vi "Check DO Channel Settings.vi"(8 "error in":errorcluster, 9 "read channel settings":T1[](array[typedef]), 10 "initial channel settings":T1[](array[typedef]), 11 "TestCase in":refnum<class "TestCase.lvclass">) -> (0 "error out":errorcluster, 3 "TestCase out":refnum<class "TestCase.lvclass">)   [LabVIEW 2017, in "Module Test.lvclass"]
uses:
  Module Test Classes/Module Test.lvclass
  Scripting/Modules/Mode Classes/Controls/digital channel settings.ctl
  <vilib>/addons/_JKI Toolkits/VI Tester/TestCase.llb/TestCase.lvclass
  Scripting/Scan Engine Scripting.lvlib
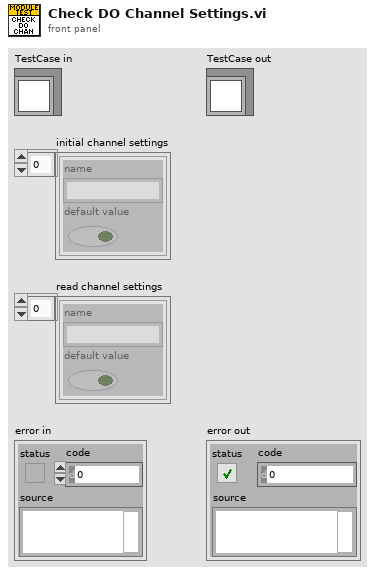
[diagram p1: front panel]
types:
  T1 = typedef "Scan Engine Scripting.lvlib/digital channel settings.ctl" = cluster{"name":string, "default value":bool}
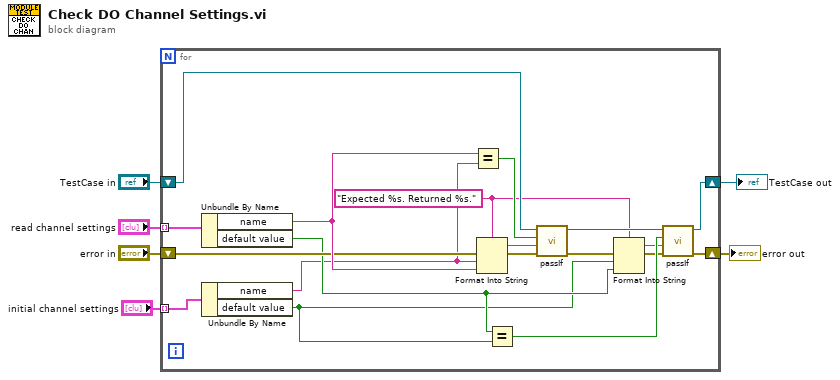
[diagram p0: block diagram]
diagram:
  n1 = for {
    tunnel: "read channel settings" -> [w24] mode=indexing
    tunnel: "initial channel settings" -> [w25] mode=indexing
    shift-right: [w16] -> w3
    shift-left: "TestCase in" -> [w23]
    shift-right: [w12] -> w1
    shift-left: "error in" -> [w20]
    w11 = "Expected %s. Returned %s." ("format string")
    n2 = Unbundle By Name(w24) -> ("name"=w21:string, "default value"=w15:bool)
    n3 = Unbundle By Name(w25) -> ("name"=w7:string, "default value"=w10:bool)
    n4 = Equal?(x=w21, y=w7) -> (x = y?=w22:bool)
    n5 = Format Into String(format string=w11, error in=w20, w7, w21) -> (resulting string=w9:string, error out=w19:errorcluster)  [unwired: 1 in]
    n6 = Equal?(x=w15, y=w10) -> (x = y?=w17:bool)
    n7 = call-dynamic "passIf.vi"("error in (no error)"=w19, "message (\"\")"=w9, "pass"=w22, "TestCase in"=w23) -> ("error out"=w14:errorcluster, "TestCase out"=w18:refnum<class "TestCase.lvclass">)  [unwired: 6 in]
    n8 = Format Into String(format string=w11, error in=w14, w10, w15) -> (resulting string=w8:string, error out=w13:errorcluster)  [unwired: 1 in]
    n9 = call-dynamic "passIf.vi"("error in (no error)"=w13, "message (\"\")"=w8, "pass"=w17, "TestCase in"=w18) -> ("error out"=w12:errorcluster, "TestCase out"=w16:refnum<class "TestCase.lvclass">)  [unwired: 6 in]
  }
  "TestCase out" <- w3
  "error out" <- w1
